vi "Xbox Remote Diagnostic.vi"() -> ()   [LabVIEW 2009]
uses:
  Remote Control/Motor Command.ctl
  Remote Control/Control Message.ctl
  Remote Control/Message Type.ctl
  UDP Lib/UDP Network Location.ctl
panel:
  in  "stop":bool
  in  "Pause Motors":bool
  out "MC Init":bool=TRUE
  out "Error Code Out":i32
  out "Motor Command":T1
  out "HB":bool
  out "error out":errorcluster
  out "Tablet Network Location":T2={"IP Address"="192.168.1.124", "Port"=50000}
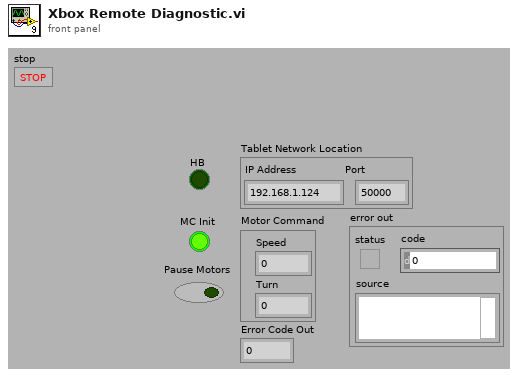
[diagram p1: front panel]
types:
  T1 = typedef "Motor Command.ctl" = cluster{"Speed":i16, "Turn":i16}
  T2 = typedef "UDP Network Location.ctl" = cluster{"IP Address":string, "Port":u16}
  T3 = typedef "UDP Base.ctl" = cluster{"UDP Session":refnum<k16>, "UDP Socket Params":T4}
  T4 = typedef "UDP Socket Params.ctl" = cluster{"Local Port":u16, "Read Timeout":i32, "Write Timeout":i32}
  T5 = typedef "Message Type.ctl" = enum16{"Motor Command", "Debug Data"}
  T6 = typedef "Control Message.ctl" = cluster{"Motor Command":T1, "Time Stamp":timestamp, "Remote  Control/!Autonomous":bool, "Send Debug Data?":bool}
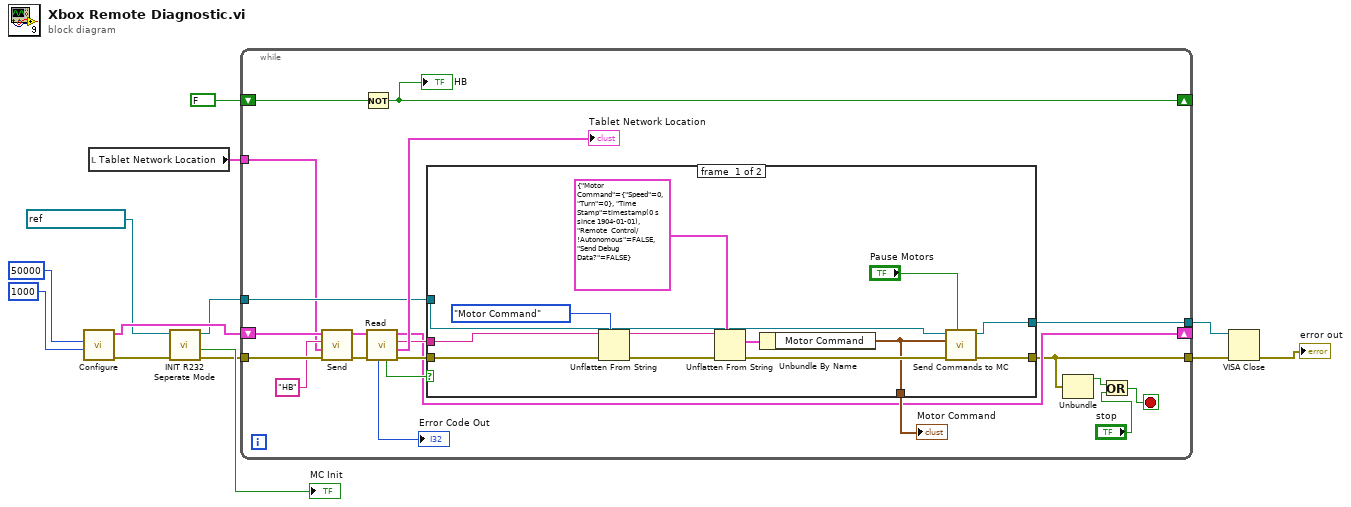
[diagram p0: block diagram]
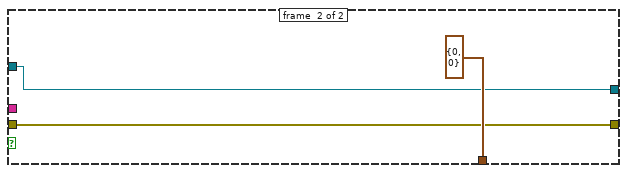
[diagram p2: hidden frame]
diagram:
  n1 = call "Configure.vi"("Read Timeout"=1000, "Local Port"=u16 50000) -> ("error out"=w8:errorcluster, "UDP Base out"=w13:T3)  [unwired: 8 in]
  n2 = local read "Tablet Network Location"() -> (w1:T2)
  n3 = call "INIT R232 Seperate Mode.vi"("error in (no error)"=w8, "MC VISA resource in"=refnum<visa-resource-name> "ASRL1::INSTR") -> ("MC error out"=w7:errorcluster, "MC Init Complete"=→"MC Init":bool, "MC VISA resource  out"=w6:refnum<visa-resource-name>)  [unwired: 7 in]
  n4 = while {
    tunnel: w7 -> [w16]
    shift-right: [w28] -> _
    shift-left: FALSE ("Timeout") -> [w29]
    shift-right: [w26] -> _
    shift-left: w13 -> [w19]
    tunnel: w6 -> [w25]
    tunnel: [w21] -> w3
    tunnel: [w24] -> w2
    tunnel: w1 -> [w14]
    stop <- w23 stop-if-true
    n5 = call "Send.vi"("error in (no error)"=w16, "Destination Location"=w14, "Send Data"="HB", "UDP Base in"=w19) -> ("error out"=w17:errorcluster, "UDP Base out"=w18:T3)  [unwired: 5 in, 1 out]
    n6 = Not(x=w29) -> (.not. x?=w28:bool)
    "HB" <- w28
    n7 = call "Read.vi"("error in (no error)"=w17, "UDP Base in"=w18) -> ("error out"=w31:errorcluster, "Network Location"=→"Tablet Network Location":T2, "Receive Data"=w32:string, "UDP Base out"=w26:T3, "Timeout"=w33:bool, "Error Code Out"=→"Error Code Out":i32)  [unwired: 4 in]
    n8 = case shown="False" w33 {
      tunnel: w32 -> [w45 _]
      tunnel: w31 -> [w44 w49]
      tunnel: [w38 T1 {"Speed"=0, "Turn"=0} ("Motor Command")] -> w30
      tunnel: [w39 w49] -> w21
      tunnel: w25 -> [w37 w48]
      tunnel: [w35 w48] -> w24
      frame #0 {
        n9 = Unflatten From String(type=Message_Type."Motor Command" ("Message Type"), binary string=w45, error in (no error)=w44) -> (rest of the binary string=w43:string, error out=w42:errorcluster)  [unwired: 2 in, 1 out]
        n10 = Unflatten From String(type=T6 {"Motor Command"={"Speed"=0, "Turn"=0}, "Time Stamp"=timestamp(0 s since 1904-01-01), "Remote  Control/!Autonomous"=FALSE, "Send Debug Data?"=FALSE} ("Control Cluster"), binary string=w43, error in (no error)=w42) -> (value=w46:T6, error out=w40:errorcluster)  [unwired: 2 in, 1 out]
        n11 = Unbundle By Name(w46) -> ("Motor Command"=w38:T1)
        n12 = call "Send Commands to MC.vi"("MC refrence in"=w37, "Motor Command"=w38, "error in"=w40, "Pause Motors"="Pause Motors") -> ("MC refrence out"=w35:refnum<visa-resource-name>, "error out"=w39:errorcluster)  [unwired: 4 in, 1 out]
      }
      frame #1 {
      }
    }
    "Motor Command" <- w30
    n13 = Unbundle(w21) -> ("status"=w20:bool)  [unwired: 2 out]
    n14 = Or(x=w20, y="stop") -> (x .or. y?=w23:bool)
  }
  n15 = VISA Close(VISA resource name=w2, error in (no error)=w3) -> (error out=→"error out":errorcluster)
